vi "Check TIFF file.vi"(8 "error in (no error)":errorcluster, 9 "Expected TIFF slices":i32, 10 "TIFF File path":path, 11 "TomoConversion in":refnum<class "TomoConversion.lvclass">) -> (0 "error out":errorcluster, 2 "is fine?":bool, 3 "TomoConversion out":refnum<class "TomoConversion.lvclass">)   [LabVIEW 2012, in "TomoConversion.lvclass"]
uses:
  TomoConversion.lvclass
  dependencies/LabTIFF/LabTIFF/Opening Purpose.ctl
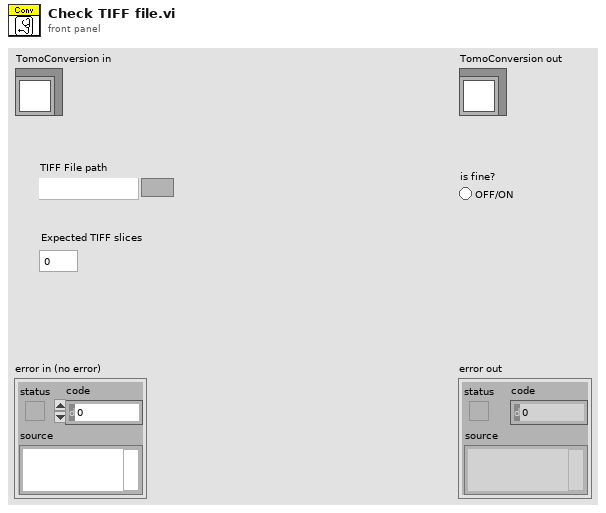
[diagram p1: front panel]
types:
  T1 = typedef "Opening Purpose.ctl" = enum16{"Read", "Write"}
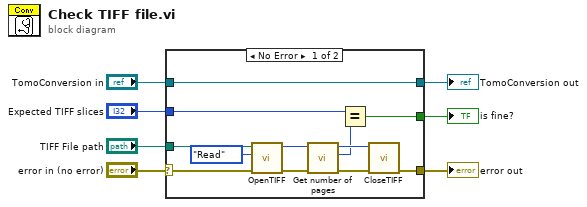
[diagram p0: block diagram]
diagram:
  n1 = case shown="No Error" "error in (no error)" {
    selector: "error in (no error)" -> [w18 w21]
    tunnel: [w12 w21] -> w6
    tunnel: [w19 w20] -> w4
    tunnel: "TomoConversion in" -> [w19 w20]
    tunnel: "TIFF File path" -> [w17 _]
    tunnel: "Expected TIFF slices" -> [w10 _]
    tunnel: [w8 _] -> w1
    frame No Error {
      n2 = call "OpenTIFF.vi"("error in (no error)"=w18, "Opening Purpose"=Opening_Purpose."Read", "File Path"=w17) -> ("error out"=w15:errorcluster, "TIFF File Ref"=w14:i32)  [unwired: 7 in]
      n3 = call "Get number of pages.vi"("error in (no error)"=w15, "TIFF File ref"=w14) -> ("error out"=w13:errorcluster, "Number of Pages"=w9:i32, "TIFF File ref out"=w11:i32)  [unwired: 7 in]
      n4 = Equal?(x=w10, y=w9) -> (x = y?=w8:bool)
      n5 = call "CloseTIFF.vi"("error in (no error)"=w13, "TIFF File Ref"=w11) -> ("error out"=w12:errorcluster)  [unwired: 9 in]
    }
    frame Error {
    }
  }
  "error out" <- w6
  "TomoConversion out" <- w4
  "is fine?" <- w1
